vi "save new configs.vi"(0 "Working Directory":path, 2 "Max File Size (Bytes)":i32=1048576, 3 "Write To File":bool, 5 "error in":errorcluster, 6 "Data File Prefix":string="data", 8 "Scan Rate (Hz)":dbl=500.0 format="%.3f", 9 "Interval (ms)":u32=500, 10 "Graph History":i32=1000 min=0, 11 "Resolution":u8, 12 "# Channels":i32=4, 13 "SettlingFactor":u8, 17 "Channel Setup":T1={"+Ch"=["0", "1", "2", "3", "4", "5", "6", "7"], "-Ch"=["199", "199", "199", "199", "199", "199", "199", "199"], "Ranges"=[0, 0, 0, 0, 0, 0, 0, 0], "Scaling Equation"=["y=v0", "y=v1", "y=v2", "y=v3", "y=v4", "y=v5", "y=v6", "y=v7"], "Graph?"=[]} {"Ranges" items=["LJ_rgBIP10V", "LJ_rgBIP5V", "LJ_rgUNI5V", "LJ_rgUNI2P5V", "LJ_rgUNI1P25V", "LJ_rgBIP1V", "LJ_rgUNIP625V", "LJ_rgBIPP1V", "LJ_rgBIPP01V"]}) -> (14 "Working Directory Out":path, 19 "error out":errorcluster)   [LabVIEW 2020]
uses:
  Instance           1 24Saved   save new configs .vi
panel:
  in  "Disable Scaling":bool
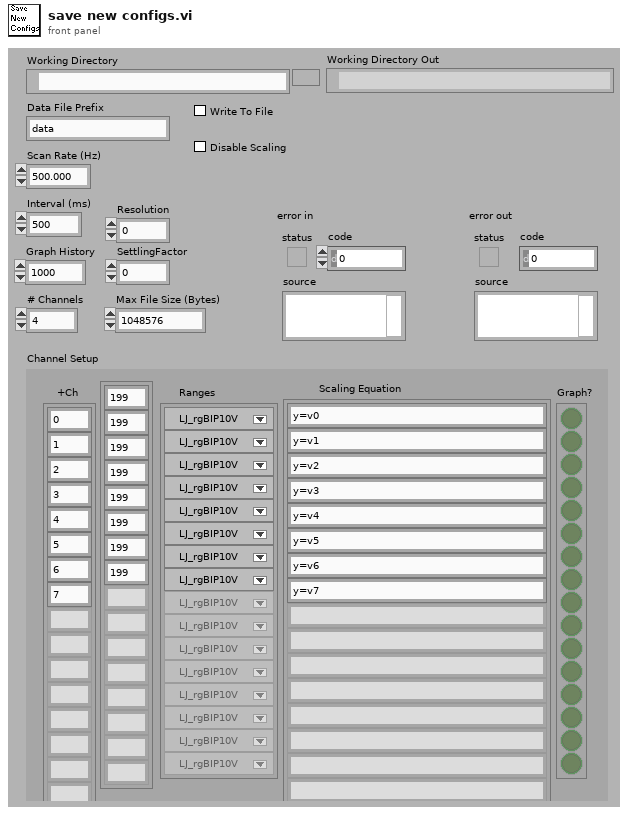
[diagram p1: front panel]
types:
  T1 = cluster{"+Ch":string[], "-Ch":string[], "Ranges":u16[], "Scaling Equation":string[], "Graph?":bool[]}
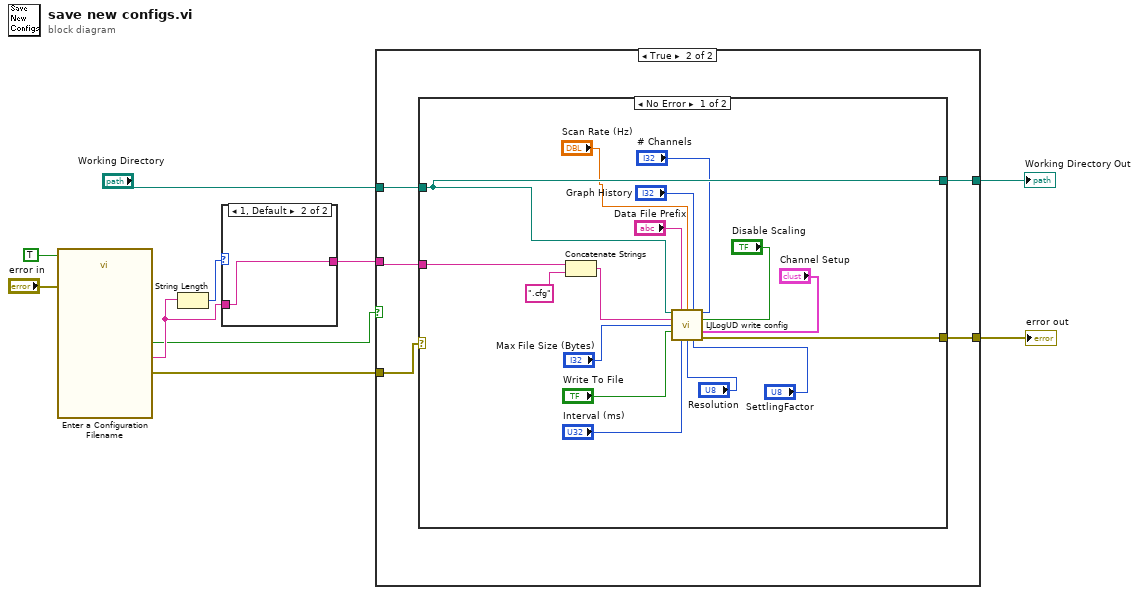
[diagram p0: block diagram]
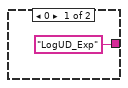
[diagram p4: hidden frame]
diagram:
  n1 = call "Enter a Configuration Filename"("Enable"=TRUE, "error in (no error)"="error in") -> ("Filename"=w3:string, "OK"=w1:bool, "error out"=w5:errorcluster)  [unwired: 15 in]
  n2 = String Length(string=w3) -> (length=w4:i32)
  n3 = case shown="1, Default" w4 {
    tunnel: w3 -> [_ w12]
    tunnel: ["LogUD_Exp" w12] -> w2
    frame 0 {
    }
    frame 1, Default {
    }
  }
  n4 = case shown="True" w1 {
    tunnel: [w13 w19] -> w10
    tunnel: [w14 w18] -> w9
    tunnel: "Working Directory" -> [w14 w17]
    tunnel: w5 -> [w13 w16]
    tunnel: w2 -> [_ w15]
    frame False {
    }
    frame True {
      n5 = case shown="No Error" w16 {
        selector: w16 -> [_ w37]
        tunnel: [w34 w37] -> w19
        tunnel: [w35 w36] -> w18
        tunnel: w17 -> [w35 w36]
        tunnel: w15 -> [w21 _]
        frame No Error {
          n6 = Concatenate Strings(w21, ".cfg" ("string")) -> (w30:string)
          n7 = call "LJLogUD write config.vi"("Working Directory"=w35, "Data File Prefix"="Data File Prefix", "Scan Rate (Hz)"="Scan Rate (Hz)", "Graph History"="Graph History", "# Channels"="# Channels", "filename"=w30, "Disable Scaling"="Disable Scaling", "Max File Size (Bytes)"="Max File Size (Bytes)", "Write To File"="Write To File", "Channel Setup"="Channel Setup", "Interval (ms)"="Interval (ms)", "Resolution"="Resolution", "SettlingFactor"="SettlingFactor") -> ("error out"=w34:errorcluster)  [unwired: 2 in]
        }
        frame Error {
        }
      }
    }
  }
  "error out" <- w10
  "Working Directory Out" <- w9
